vi "SGL Array to U16 Array.vi"(11 "SGL":sgl[](array[numeric])) -> (3 "REG U16":u16[](array[numeric]))   [LabVIEW 2019, in "Modbus DataType Conversation.lvlib"]
uses:
  Modbus DataType Conversation.lvlib
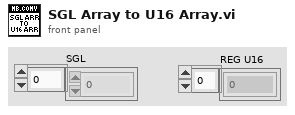
[diagram p1: front panel]
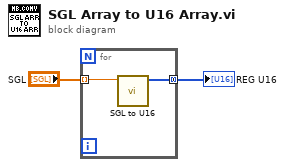
[diagram p0: block diagram]
diagram:
  n1 = for {
    tunnel: [w4] -> w2 mode=concatenating
    tunnel: "SGL" -> [w3] mode=indexing
    n2 = call "SGL to U16.vi"("SGL"=w3) -> ("U16"=w4:u16[])  [unwired: 10 in]
  }
  "REG U16" <- w2
